vi "AsyncExample.vi"() -> ()   [LabVIEW 2019, in "MicronTemplateAPIs.lvlib" / "MicronTemplateAPIs.lvclass"]
uses:
  MicronTemplateAPIs.lvclass
  vi.lib/Micron/gRPC/Client/Typedefs/AsyncMessageResponse.ctl
  vi.lib/Micron/gRPC/Client/Generated/MicronGRPCGeneratedClient/RPC Messages/micronGrpc_MessageRequest.ctl
  vi.lib/Micron/gRPC/Client/Generated/MicronGRPCGeneratedClient/RPC Messages/micronGrpc_MessageReply.ctl
  vi.lib/Micron/gRPC/Client/Generated/MicronGRPCGeneratedClient/RPC Messages/micronGrpc_MessageReply_Status.ctl
  vi.lib/Micron/Base/Client/Typedefs/ServiceDetails.ctl
  78909296-a6b7-4131-b351-69347a1d12dc.vi
  9ceadd3c-745e-4cc0-becc-c9896ef65399.vi
  <vilib>/SLL Toolkit/SLL File IO/SLL File IO.lvlib
  vi.lib/Micron/Base/Client/MicronClient.lvclass
  vi.lib/Micron/gRPC/Client/Generated/MicronGRPCGeneratedClient/MicronGRPCGeneratedClient.lvlib
  vi.lib/Micron/gRPC/Client/MicronGRPCClient.lvclass
panel:
  in  "Collect Response?":bool
  out "Responses":T1[](array[typedef])
  in  "Repeat Count":i32=10
  in  "Connection Type":enum32{"Start New", "Connect Existing"}(tab)
  in  "Mode":string(combo)="Default"
  in  "Path":path
  in  "Port":i32=50051
  in  "ServiceID":string="micron-1"
  in  "UI":string(combo)="show"
  in  "Connection String":string="localhost:50051"
  out "error out":errorcluster
  in  "Command":string="Hello Micron!"
  in  "Payload":string="An Open Source Microservice Architecture on top of gRPC from https://github.com/KarthikAbiram/Micron"
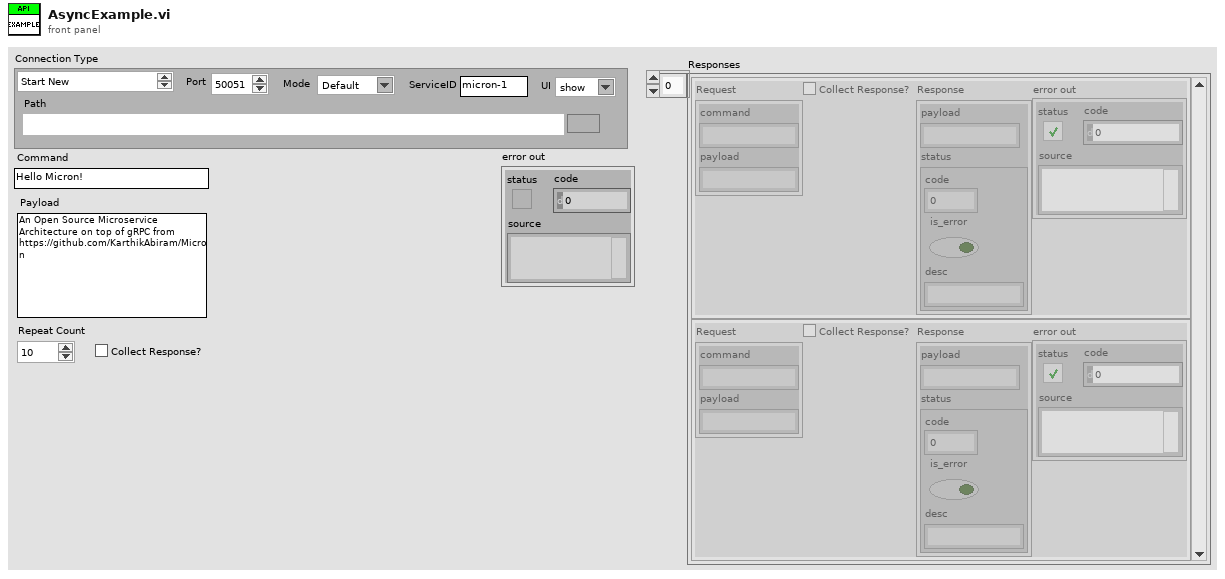
[diagram p1: front panel]
types:
  T1 = typedef "MicronGRPCClient.lvclass/AsyncMessageResponse.ctl" = cluster{"Request":T2, "Collect Response?":bool, "Response":T3, "error out":errorcluster}
  T2 = typedef "MicronGRPCGeneratedClient.lvlib/micronGrpc_MessageRequest.ctl" = cluster{"command":string, "payload":string}
  T3 = typedef "MicronGRPCGeneratedClient.lvlib/micronGrpc_MessageReply.ctl" = cluster{"payload":string, "status":T4}
  T4 = typedef "MicronGRPCGeneratedClient.lvlib/micronGrpc_MessageReply_Status.ctl" = cluster{"code":i32, "is_error":bool, "desc":string}
  T5 = typedef "MicronClient.lvclass/ServiceDetails.ctl" = cluster{"Micron Path":path, "Network":string, "ServiceID":string, "Port":i32, "FullyQualifiedName":string, "UI":string, "Args":string, "Mode":string}
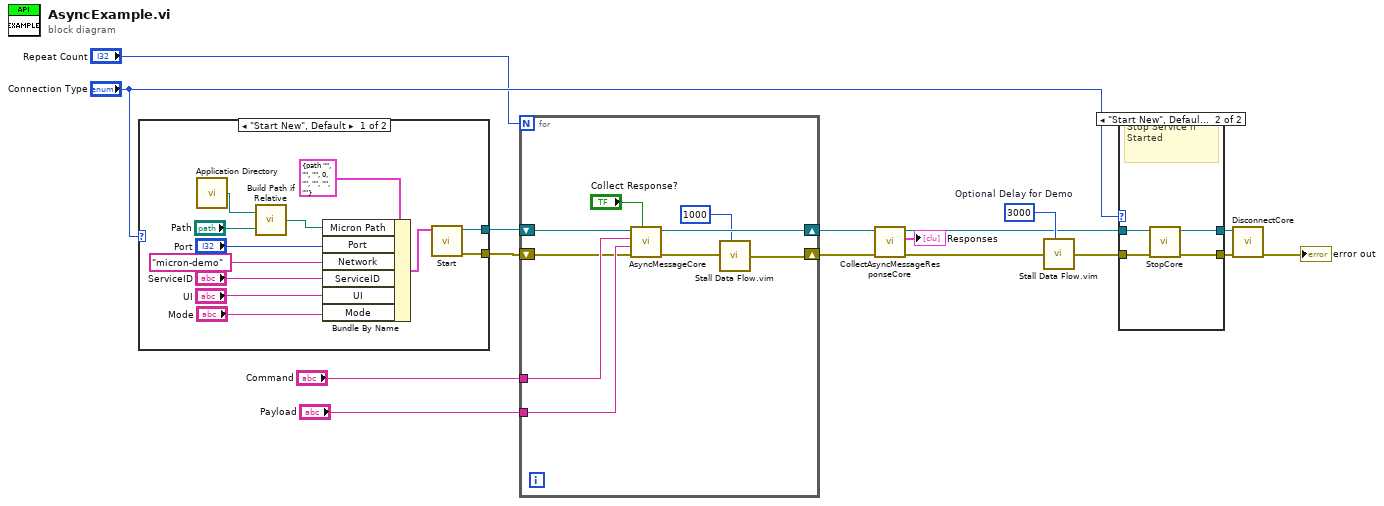
[diagram p0: block diagram]
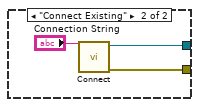
[diagram p3: hidden frame]
diagram:
  w7 = u32 3000  # Optional Delay for Demo
  n1 = case shown="\"Start New\", Default" "Connection Type" {
    tunnel: [w28 w31] -> w13
    tunnel: [w27 w30] -> w12
    frame "Start New", Default {
      n2 = call <vilib>:"Application Directory.vi"() -> ("Application Directory"=w21:path)
      n3 = call <vilib>:"Build Path if Relative.vi"("Relative or Absolute Path"="Path", "Base Path"=w21) -> ("Path Out"=w22:path)
      n4 = Bundle By Name(cluster=T5 {"Micron Path"=path "", "Network"="", "ServiceID"="", "Port"=0, "FullyQualifiedName"="", "UI"="", "Args"="", "Mode"=""} ("Service Details"), "Micron Path"=w22, "Port"="Port", "Network"="micron-demo", "ServiceID"="ServiceID", "UI"="UI", "Mode"="Mode") -> (w25:T5)
      n5 = call "Start.vi"("Service Details"=w25) -> ("error out"=w28:errorcluster, "MicronTemplateAPIs out"=w27:refnum<class "MicronTemplateAPIs.lvclass">)  [unwired: 9 in]
    }
    frame "Connect Existing" {
      n6 = call "Connect.vi"("Connection String"="Connection String") -> ("error out"=w31:errorcluster, "MicronTemplateAPIs out"=w30:refnum<class "MicronTemplateAPIs.lvclass">)  [unwired: 9 in]
    }
  }
  n7 = for {
    N: "Repeat Count" -> [_]
    tunnel: "Payload" -> [w40]
    tunnel: "Command" -> [w39]
    shift-right: [w34] -> w5
    shift-left: w13 -> [w38]
    shift-right: [w36] -> w4
    shift-left: w12 -> [w37]
    n8 = call-dynamic "AsyncMessageCore.vi"("Collect Response?"="Collect Response?", "error in (no error)"=w38, "Payload"=w40, "Command"=w39, "GRPCClient in"=w37) -> ("error out"=w35:errorcluster, "GRPCClient out"=w36:refnum<class "MicronTemplateAPIs.lvclass">)  [unwired: 5 in]
    n9 = call "Stall Data Flow.vim"("value in"=w35, "milliseconds to wait"=u32 1000) -> ("value out"=w34:errorcluster)  [unwired: 1 out]
  }
  n10 = call-dynamic "CollectAsyncMessageResponseCore.vi"("error in (no error)"=w5, "MicronGRPCClient in"=w4) -> ("error out"=w3:errorcluster, "Responses"=→"Responses":T1[], "MicronGRPCClient out"=w2:refnum<class "MicronTemplateAPIs.lvclass">)  [unwired: 7 in]
  n11 = call "Stall Data Flow.vim"("value in"=w3, "milliseconds to wait"=w7) -> ("value out"=w8:errorcluster)  [unwired: 1 out]
  n12 = case shown="\"Start New\", Default" "Connection Type" {
    tunnel: w8 -> [w42 w46]
    tunnel: w2 -> [w41 w45]
    tunnel: [w41 w44] -> w11
    tunnel: [w42 w43] -> w10
    frame "Connect Existing" {
    }
    frame "Start New", Default {
      # "Stop Service if Started"
      n13 = call-dynamic "StopCore.vi"("error in (no error)"=w46, "MicronClient in"=w45) -> ("error out"=w43:errorcluster, "MicronClient out"=w44:refnum<class "MicronTemplateAPIs.lvclass">)  [unwired: 7 in, 1 out]
    }
  }
  n14 = call-dynamic "DisconnectCore.vi"("error in (no error)"=w10, "GRPCClient in"=w11) -> ("error out"=→"error out":errorcluster)  [unwired: 8 in, 1 out]
